vi "Fetch Multiple Record Raw Data (I16).vi"(5 "FIFO Type":enum16{"FPGA to Host FIFO (U64)", "Generic"}(ring), 7 "Timeout (s)":i32=5, 8 "error in":errorcluster, 10 "Records to Fetch":i32, 11 "FPGA VI Reference In":refnum<k20>) -> (0 "error out":errorcluster, 2 "Acquired Data":i16[](array[numeric]), 3 "FPGA VI Reference Out":refnum<k20>, 4 "Elements Remaining":u32)   [LabVIEW 2011]
uses:
  <userlib>/FlexRIO Host Library/FlexRIO Host API/Acquire/Fetch/Fetch Acquired Data (U64).vi
  <vilib>/Utility/error.llb/Error Cluster From Error Code.vi
  <vilib>/rvi/errors/niLvFpgaAdjustHostInterfaceError.vi
  <vilib>/rvi/interface/nirviReadWriteControl/nirviReadWriteControl.xnode
  NiFpgaLv.dll
  <vilib>/rvi/interface/Simulation/niFpgaSimulationCallBeginRW.vi
  <userlib>/FlexRIO Host Library/FlexRIO Host Library (User).lvlib
  <userlib>/FlexRIO Host Library/FlexRIO Host API/Utility/memnoncopy.dll
panel:
  out "Data Acquired":i16[](array[numeric])
  out "Dummy Data":i16[](array[numeric])
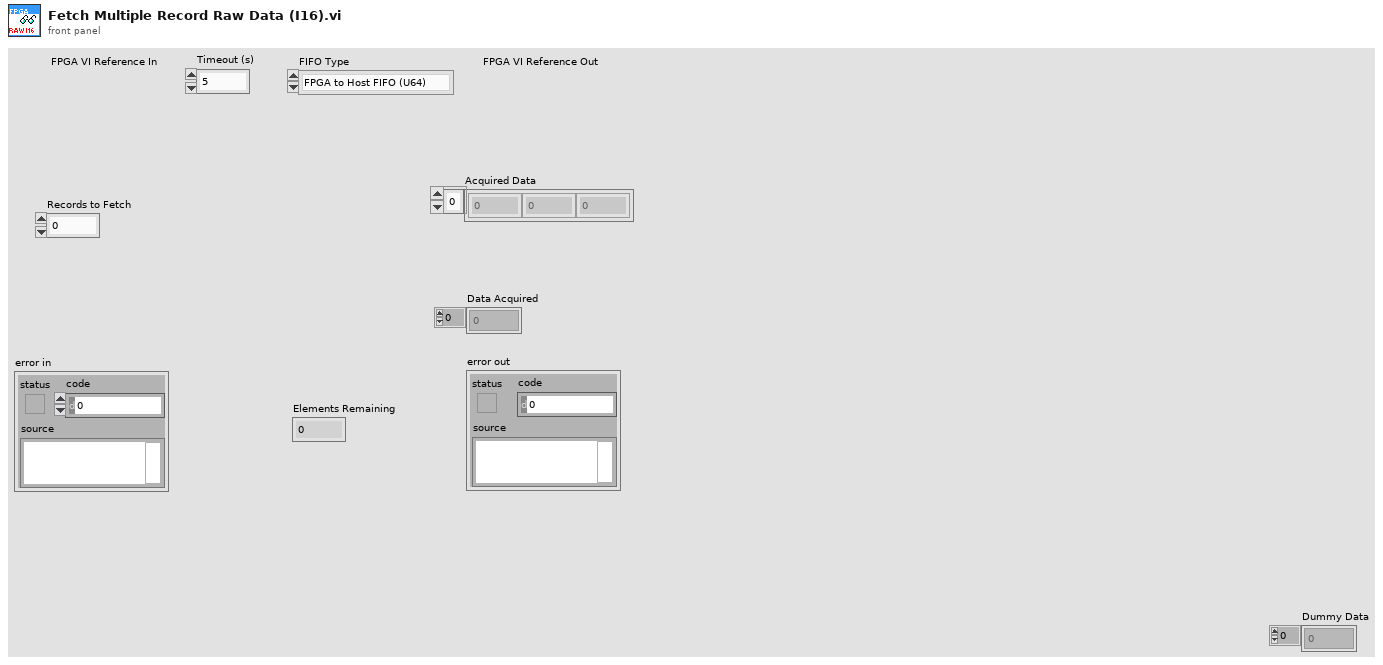
[diagram p1: front panel]
types:
  T1 = cluster{"Load Record Parameters?":bool, "Pre Trigger Samples":u16, "Samples per Record":u16, "Trigger Hold Off":u16, "Record Count":u16}
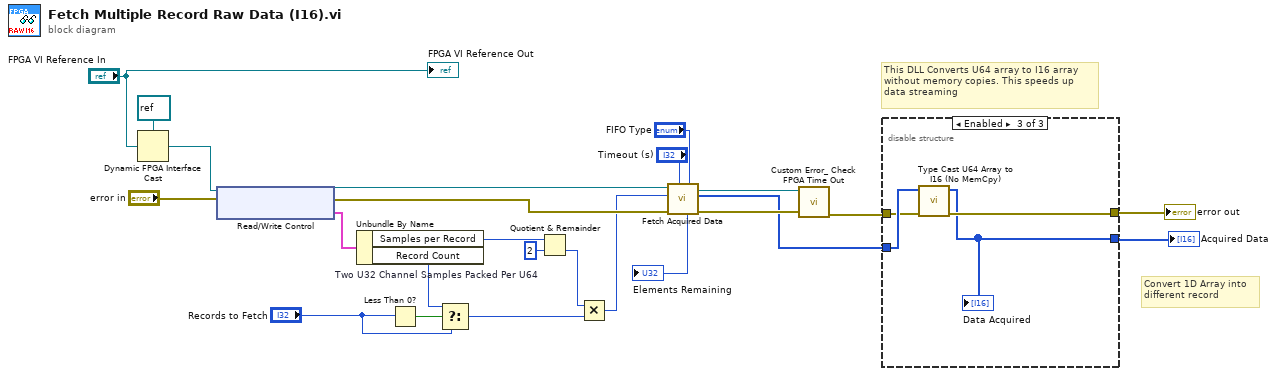
[diagram p0: block diagram]
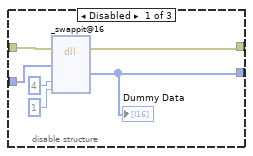
[diagram p2: hidden frame]
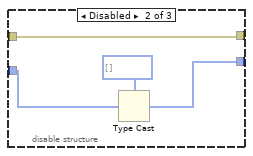
[diagram p3: hidden frame]
diagram:
  w7 = u16 2  # Two U32 Channel Samples Packed Per U64
  # "This DLL Converts U64 array to I16 array \nwithout memory copies. This speeds up \ndata streaming"
  # "Convert 1D Array into\ndifferent record"
  n1 = Dynamic FPGA Interface Cast(Session In=refnum<k20> refnum ("Type"), Type="FPGA VI Reference In") -> (Session Out=w21:refnum<k20>)
  n2 = xnode "Read/Write Control"("FPGA VI Reference In"=w21, "error in"="error in") -> ("FPGA VI Reference Out"=w16:refnum<k20>, "error out"=w15:errorcluster, "Record Parameters"=w20:T1)
  n3 = Unbundle By Name(w20) -> ("Samples per Record"=w8:u16, "Record Count"=w18:u16)
  n4 = Less Than 0?(x="Records to Fetch") -> (x < 0?=w19:bool)
  n5 = Select(t=w18, s=w19, f="Records to Fetch") -> (s? t:f=w2:i32)
  n6 = Quotient & Remainder(x=w8, y=w7) -> (floor(x/y)=w3:u16)  [unwired: 1 out]
  n7 = Multiply(x=w3, y=w2) -> (x*y=w9:i32)
  n8 = call-poly <userlib>:"Fetch Acquired Data.vi"("FIFO Type"="FIFO Type", "Timeout (s)"="Timeout (s)", "error out"=w15, "Samples"=w9, "FPGA VI Reference In"=w16) -> ("error out"=w10:errorcluster, "Data"=w4:u64[], "FPGA VI Reference Out"=w11:refnum<k20>, "Elements Remaining"=→"Elements Remaining":u32)  [unwired: 3 in]
  n9 = call <userlib>:"Custom Error_ Check FPGA Time Out.vi"("error in"=w10, "FPGA VI Reference In"=w11) -> ("error out"=w6:errorcluster)  [unwired: 8 in, 1 out]
  n10 = disable-structure shown="Enabled" {
    disable-tunnel: w4 -> [w28 w33 w38]
    disable-tunnel: w6 -> [w27 w31 w37]
    disable-tunnel: [w26 w31 w36] -> w5
    disable-tunnel: [w25 w32 w35] -> w1
    frame Disabled {
      n11 = dll-call lib="C:/Program Files (x86)/National Instruments/LabVIEW 2011/user.lib/FlexRIO Host Library/FlexRIO Host API/Utility/memnoncopy.dll" fn="_swappit@16"(error in=w27, "src"=w28, "upsize"=4, "downsize"=1) -> (error out=w26:errorcluster, "Dummy Data"=w25:i16[])  [unwired: 7 in, 1 out]
      "Dummy Data" <- w25
    }
    frame Disabled {
      n12 = Type Cast(type=i16[] [], x=w33) -> (*(type *) &x=w32:i16[])
    }
    frame Enabled {
      n13 = call <userlib>:"Type Cast U64 Array to I16 (No MemCpy).vi"("error in"=w37, "Input"=w38) -> ("error out"=w36:errorcluster, "Data Acquired"=w35:i16[])  [unwired: 8 in]
      "Data Acquired" <- w35
    }
  }
  "error out" <- w5
  "Acquired Data" <- w1
  "FPGA VI Reference Out" <- "FPGA VI Reference In"
